vi "main 0.2.vi"() -> ()   [LabVIEW 2020]
uses:
  subvi/Newport ESP301/Newport ESP301.lvlib
  subvi/sp_manip.llb/sp_manip_lib.lvlib
  subvi/sp_manip.llb/tcp_gateway.lvlib
  <vilib>/Utility/file.llb/Write Delimited Spreadsheet (DBL).vi
  subvi/PHOIBOS/DEFINITIONS/DEF_dev_type.ctl
  subvi/PHOIBOS/DEFINITIONS/DEF_dev_state.ctl
  <vilib>/Utility/file.llb/Write Delimited Spreadsheet (I64).vi
panel:
  out "state":T1 items=["Off"=-1, "Standby"=0, "On"=1]
  in  "BasePath 2":path=path "Z:/PESdata"
  out "ESP_con?":bool caption="ESP301"
  out "phoib_con?":bool caption="PHOIBOS"
  out "manip_con?":bool caption="manipulator"
  out "cam_con?":bool caption="camera"
  in  "main_close":bool
  in  "Tab Control":enum32{"Live", "Measure", "Settings", "Devices"}(tab)=enum."Devices"
  out "cam_burst_progress":u8(slide) scale=0.0..200.0
  in  "cam_burstnr":u32 max=1000
  in  "cam_burst":bool
  in  "ESP_delta":dbl
  in  "ESP_+ 2":bool
  in  "ESP_+":bool
  in  "ESP_go":bool
  in  "ESP_dest_t":dbl caption="Delay"
  in  "ESP_dest":dbl caption="Position"
  in  "ESP_set_t0":bool
  in  "phoib_I_6s":dbl=3200.0
  in  "phoib_I_5s":dbl=1400.0
  in  "phoib_I_4s":dbl=4.2
  in  "phoib_I_3s":dbl
  in  "phoib_I_2s":dbl=35.0
  in  "phoib_I_1s":dbl=21.9
  in  "phoib_standby":bool
  in  "phoib_set":bool
  out "phoib_I_6":dbl caption="Screen Voltage"
  out "phoib_I_5":dbl caption="Detctor Voltage"
  out "phoib_I_4":dbl caption="Work Function"
  out "phoib_I_3":dbl caption="Coil Current"
  out "phoib_I_2":dbl caption="Pass Energy"
  out "phoib_I_1":dbl caption="Kinetic Energy"
  out "CCD temp [°C]":i32=-13
  out "electronics temp [°C]":i32=30
  out "Saved Positions":string[][](table)=[["ertwertwert", "-2.299945", "-2.030214", "38.900024", "50.000762", "0.000887", "-97.998082"], ["uztgugt", "-14.999451", "-13.638894", "442.380066", "13.998380", "-1.893758", "-76.305838"], ["asdf", "-14.999451", "-13.638894", "442.380066", "13.998380", "-1.893758", "-76.305838"], ["test3", "-14.999451", "-13.638894", "441.380066", "13.998380", "-1.893758", "-76.305838"]]
  in  "Save Pos":bool
  in  "Load":bool
  in  "Delete":bool
  in  "ManipRel":dbl=1.0
  in  "ManipRel +":bool
  in  "ManipRel -":bool
  in  "manip.rel.select":enum32{"x", "y", "z", "polar", "tilt", "azimut"}(radio)=enum."polar"
  in  "Move Abs":bool
  in  "stop manip":bool
  in  "dest":dbl[](array[numeric])=[0.007141549166819264, -0.009888298846365134, 431.30615234375, 89.00040512814502, 1.109125024699864, -227.9162918846475] caption="destinations" format="%#.5g"
  out "names":string[](array[string])=["x", "y", "z", "polar", "tilt", "azimut"]
  out "pos":dbl[](array[numeric])=[0.007141549166819264, -0.009888298846365134, 431.30615234375, 89.00040512814502, 1.109125024699864, -227.9162918846475] caption="positions" format="%.5f"
  out "Intensity Graph":u16[][](graph)
  in  "Exposure [ms]":u32=20
  in  "Mode":T2(ring)=enum."WideAngleMode"
  in  "VoltageRange":enum16{"3.5kV", "1.5kV", "400V", "100V", "10V"}(ring)=enum."400V"
  out "ESP_pos":dbl caption="Position"
  out "ESP_delay":dbl caption="Delay"
  in  "ESP_t0":dbl caption="Time Zero @"
  in  "V binning":u16(ring)=2 items=["X 1", "X 2", "X 4", "X 8", "X 16", "X 32", "X 64", "X 128", "X 256", "X 512", "X 1024"]
  in  "H binning":u16(ring)=2 items=["X 1", "X 2", "X 4", "X 8"]
  in  "cam_gain":bool
  out "opti_frames":dbl=25.0 caption="#steps_opti"
  out "opti_current_frame":i32=25
  out "Measurement Progress":u8(slide) scale=0.0..100.0
  out "Camera Aquisition":u8(slide) scale=0.0..100.0
  in  "Optimize":bool
  in  "OptiStepSize":dbl=-1.0 caption="Step Size"
  in  "OptiRange":dbl=25.0 caption="Range"
  in  "meas_axis":string(combo)="tilt" caption="Axis"
  in  "meas_avg":i32=60 caption="Frames2Average"
  in  "OptiCancel":bool
  out "#steps_opti":dbl=25.0
  out "current_step_opti":i32=25
  out "ETA":string
  in  "BasePath":path=path "Z:/PESdata"
  in  "Path":path=path "Z:/software/ManipulatorControl/save.txt"
  in  "ROI Bottom":i32=32
  in  "ROI Top":i32=1
  in  "ROI Right":i32=40
  in  "ROI Left":i32=1
  in  "ESP Axis":i32=1 min=1 max=3
  in  "manip_init":bool
  in  "manip_release":bool
  in  "phoib_init":bool
  in  "phoib_release":bool
  in  "ESP_init":bool
  in  "ESP_release":bool
  in  "ESP301 VISA":refnum<visa-resource-name>="COM8"
  in  "cam_boardnr":i32
  in  "cam_init":bool
  in  "cam_release":bool
  out "error out":errorcluster
  out "error out 2":errorcluster
  # "step _ of _"
  # "step _ of _"
  # "manip"
  # "phoib"
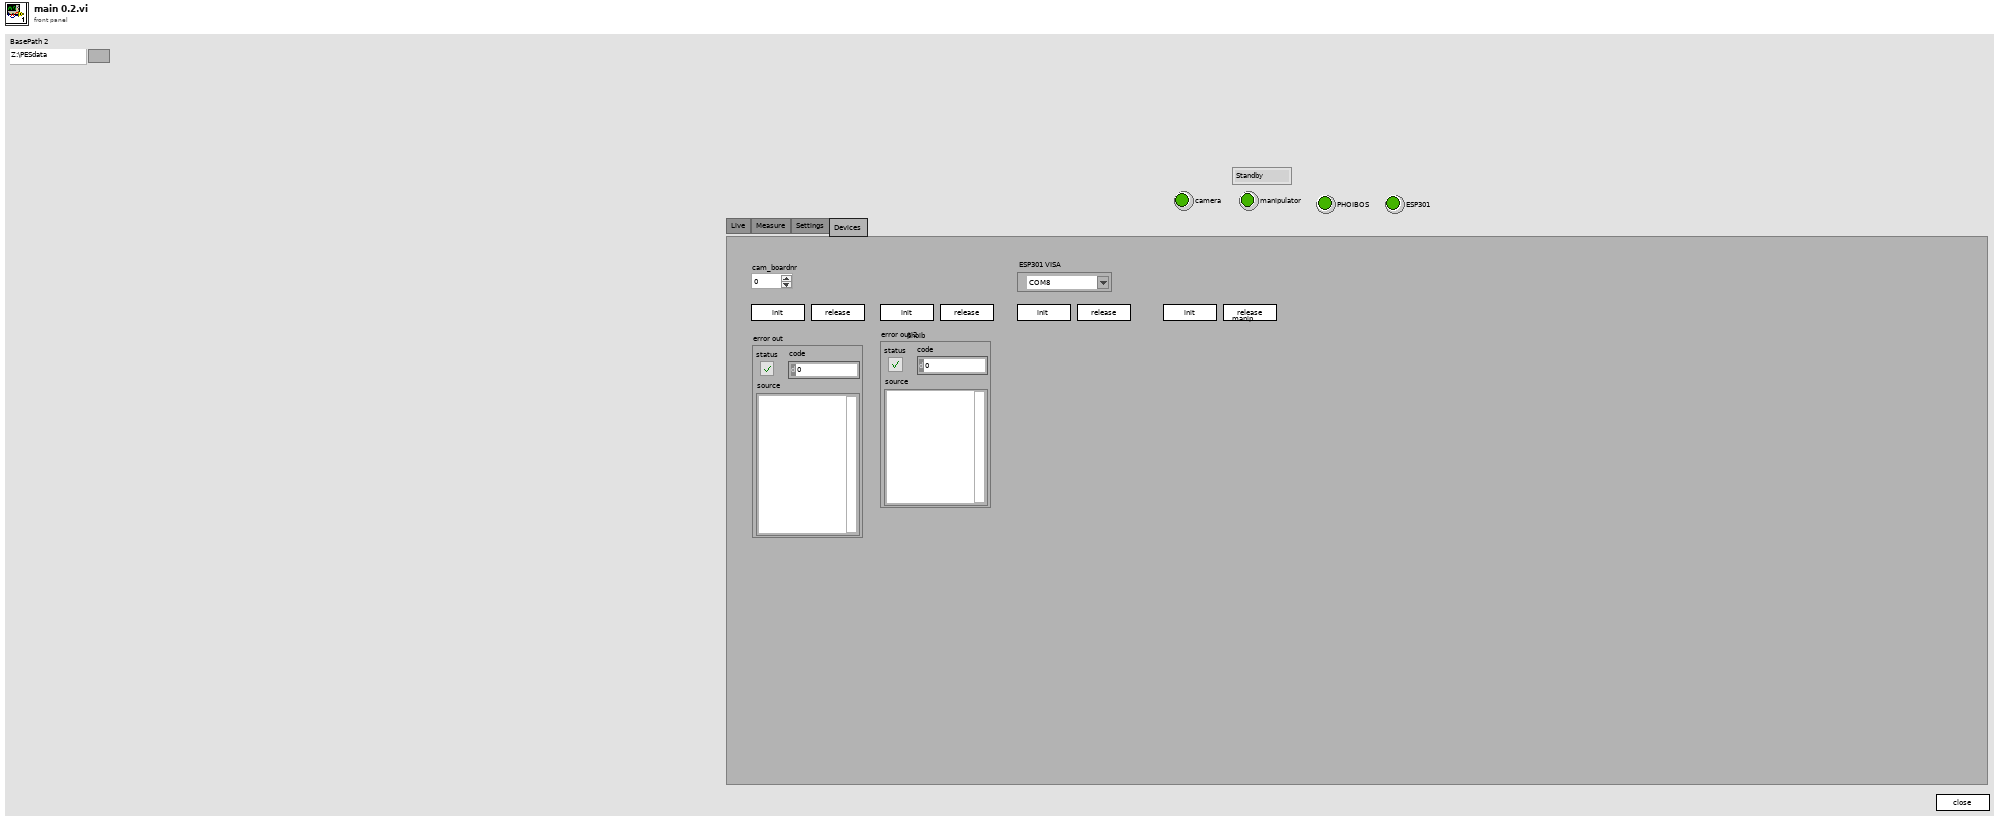
[diagram p1: front panel]
types:
  T1 = typedef "DEF_dev_state.ctl" = i32
  T2 = enum16{"HighMagnification", "MediumMagnification", "LowMagnification", "HighAngularDispersion", "MediumAngularDispersion", "LowAngularDispersion", "WideAngleMode", "LargeArea", "MediumArea", "SmallArea", "HighMagnification2", "SmallArea2", "ImagingMode"}
  T3 = cluster{"Camera type":u32, "Operating mode\nHP & QE / HS & DiCam Pro ":u32, "Frame trigger \n(High Performance and QE only)":u16, "Sequence trigger":u16, "Low Light\n(QE only)":bool, "Gain":bool, "Horzontal\nbinning":u16, "Vertical\nbinning ":u16, "ROI Left":i32, "ROI Right":i32, "ROI Top":i32, "ROI Bottom":i32}
  T4 = enum16{"open", "replace", "create", "open or create", "replace or create", "replace or create with confirmation"}
  T5 = cluster{"Axis_Name":string, "Axis_Type":string, "Axis_Position":dbl, "continous":bool, "moving":bool}[]
  T6 = cluster{"Axis_Name":string, "Axis_Type":string, "Axis_Position":dbl, "continous":bool, "moving":bool}
  T7 = typedef "DEF_dev_type.ctl" = enum32{"devA (analyzer)", "devD (detector)"}
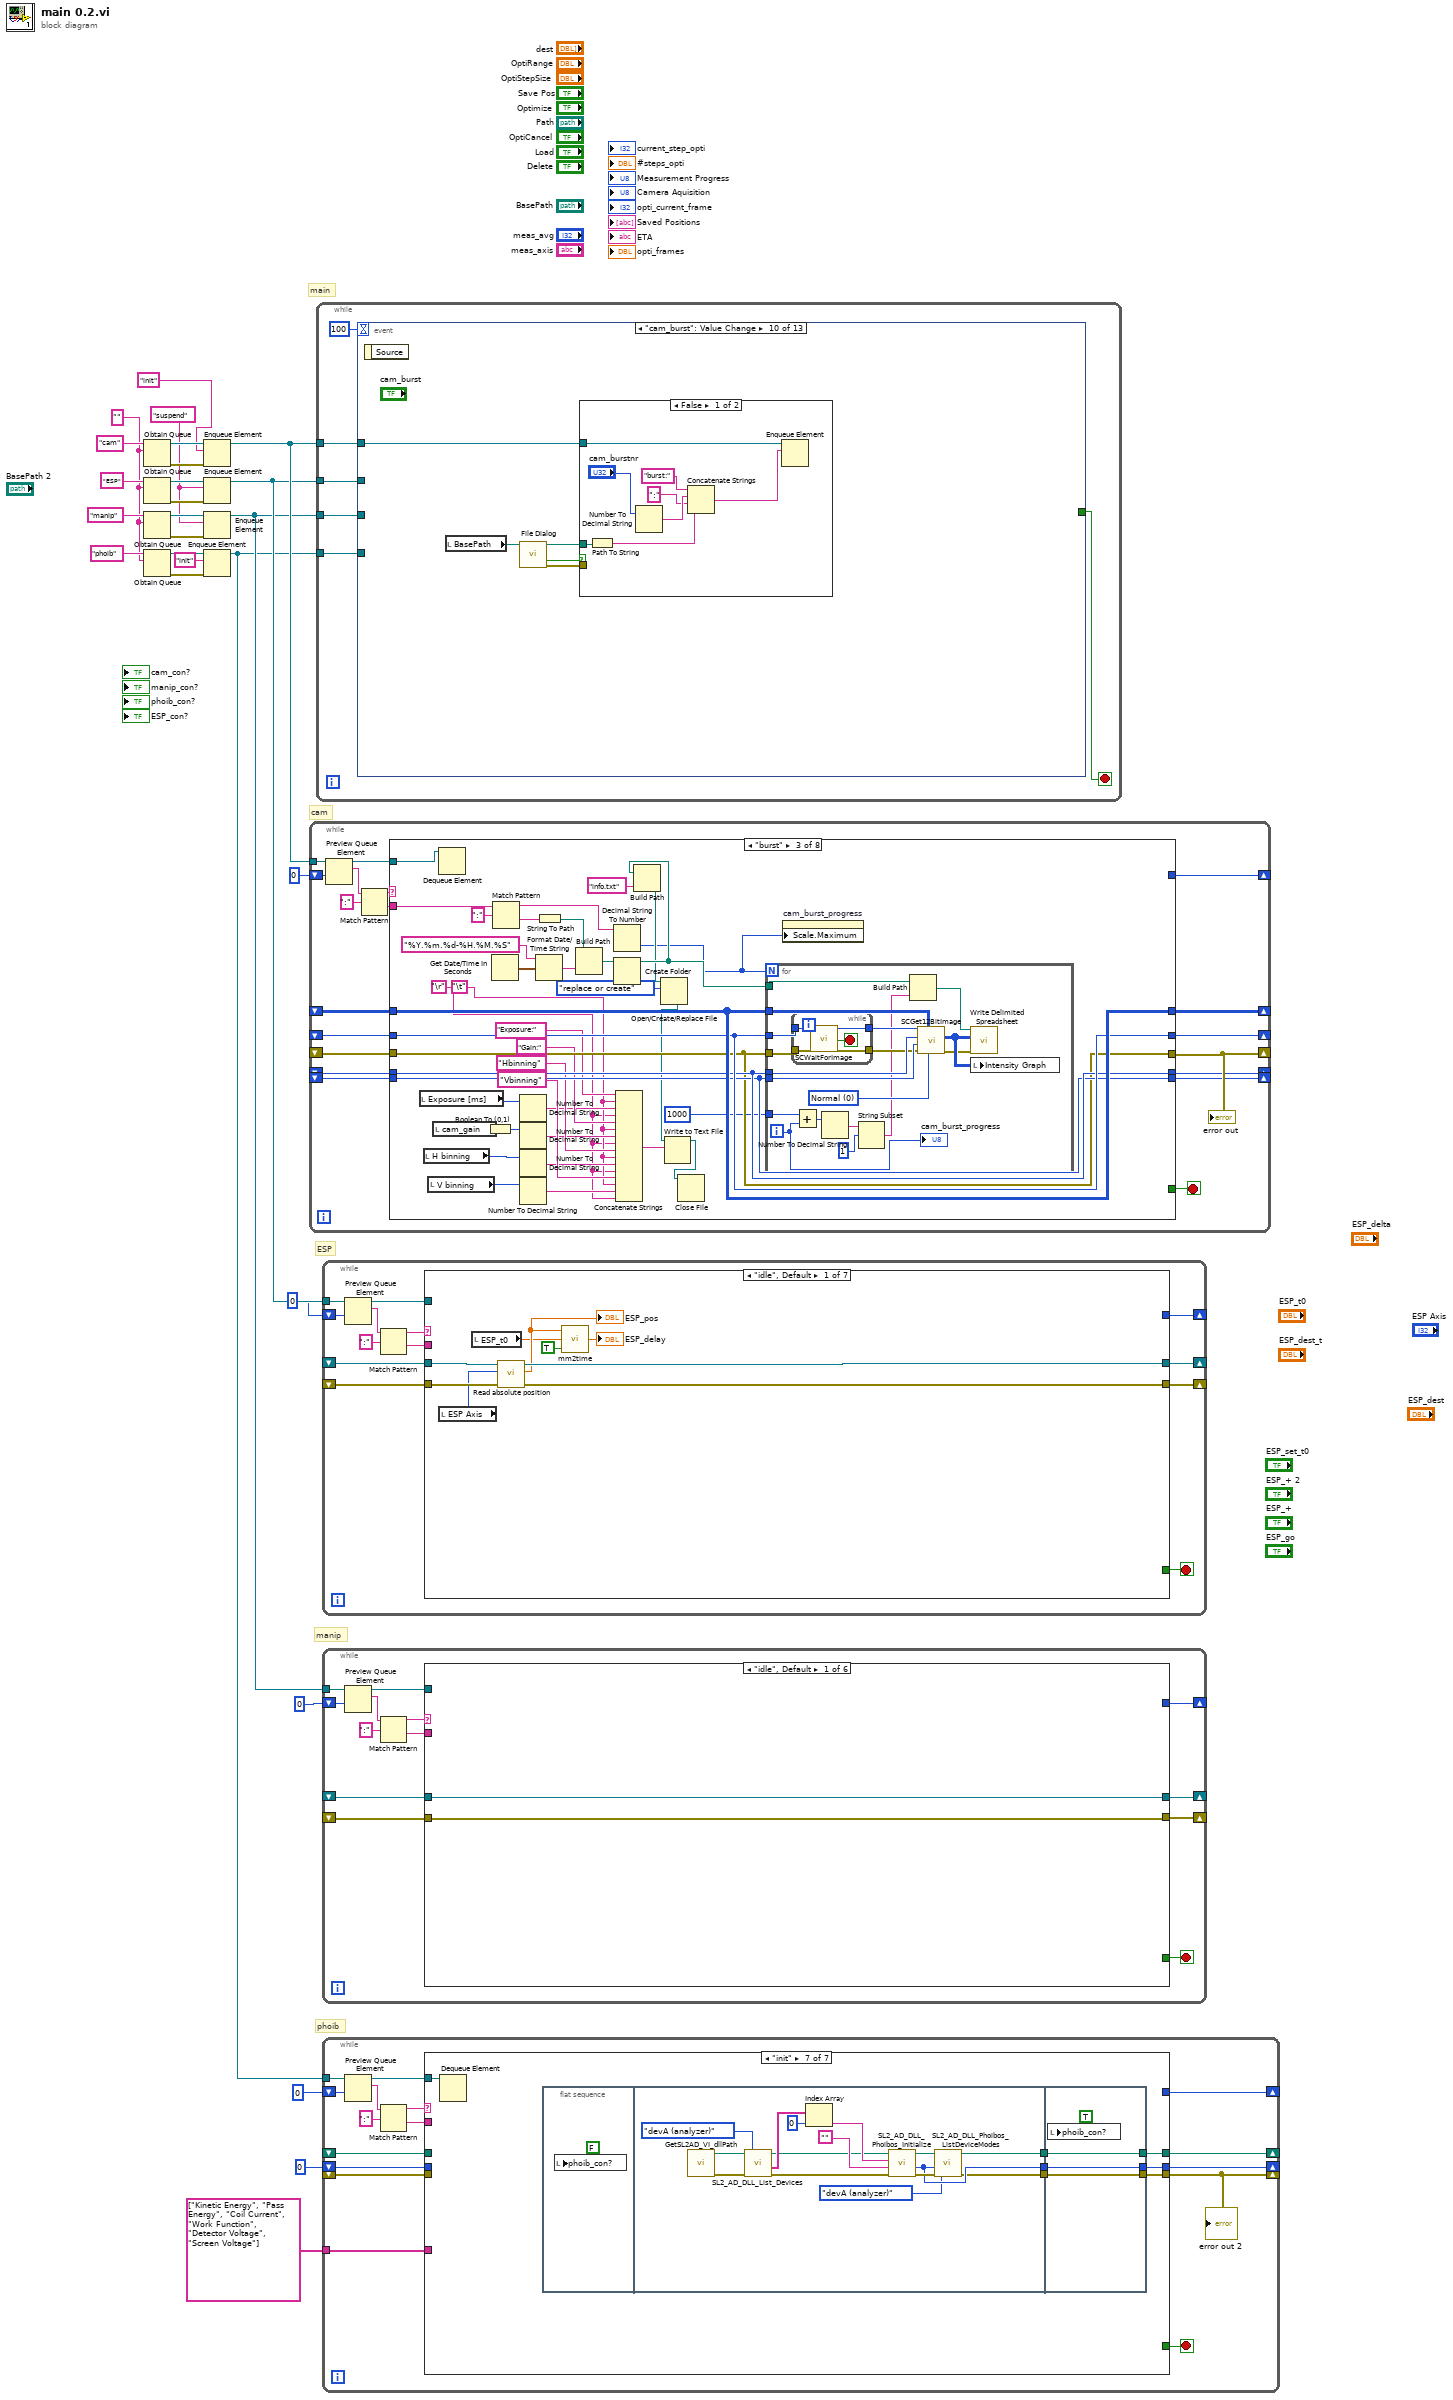
[diagram p0: block diagram]
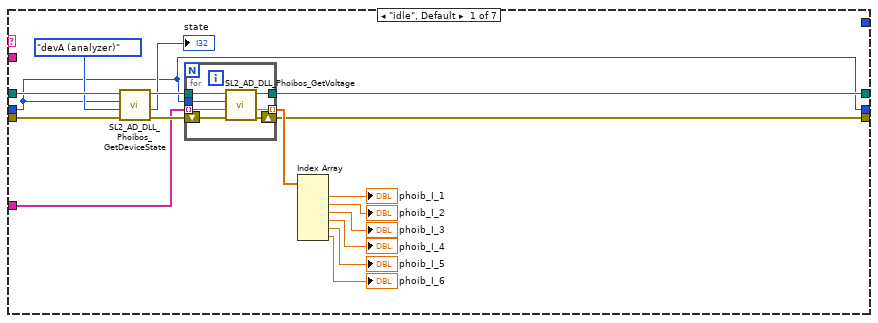
[diagram p2: hidden frame]
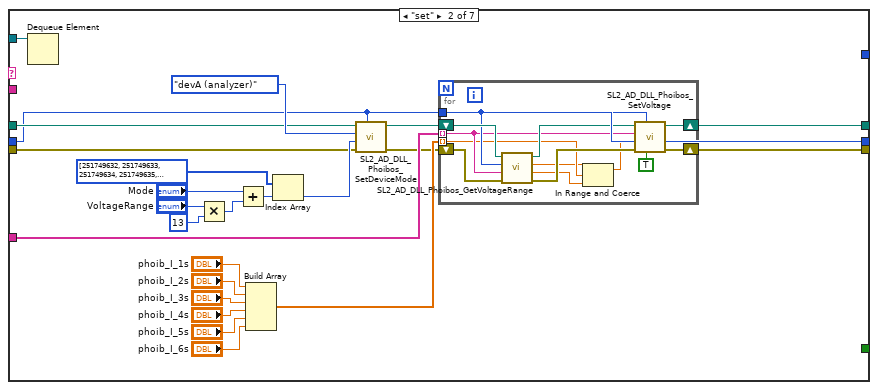
[diagram p3: hidden frame]
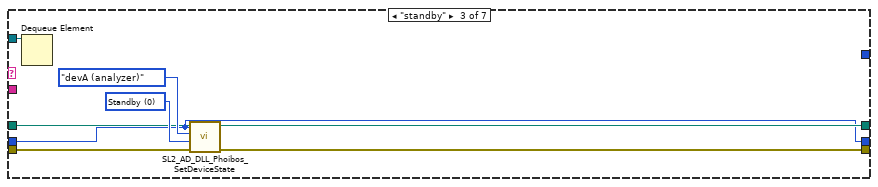
[diagram p4: hidden frame]
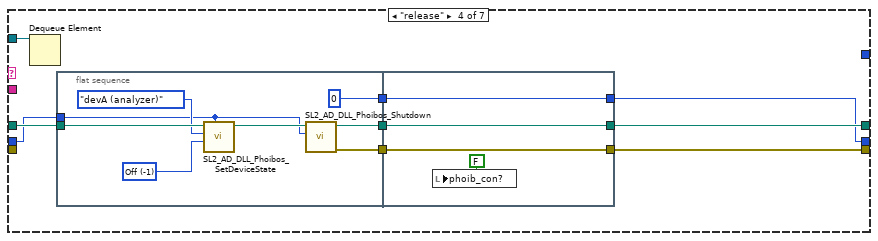
[diagram p5: hidden frame]
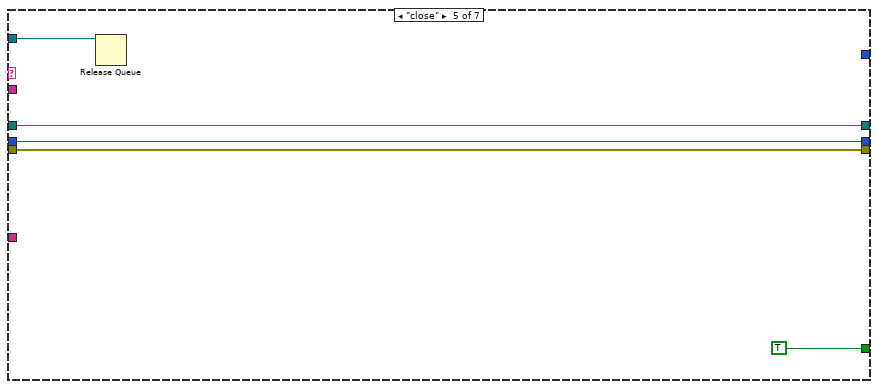
[diagram p6: hidden frame]
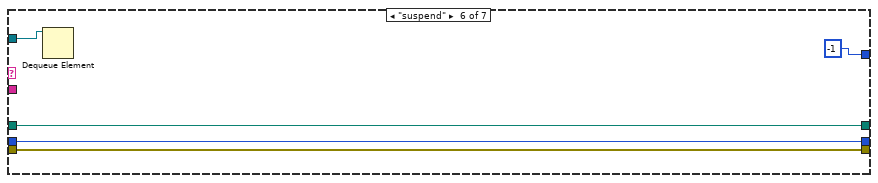
[diagram p7: hidden frame]
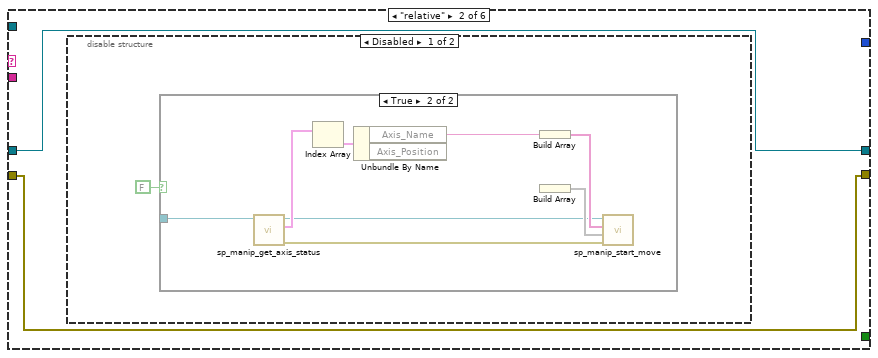
[diagram p8: hidden frame]
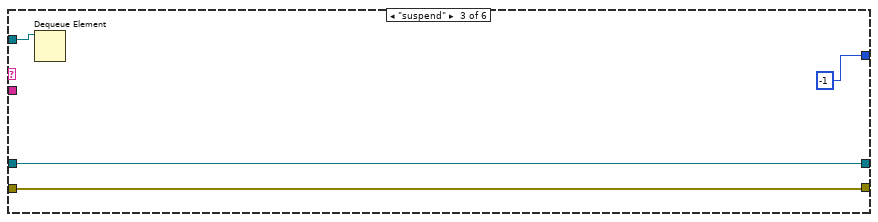
[diagram p11: hidden frame]
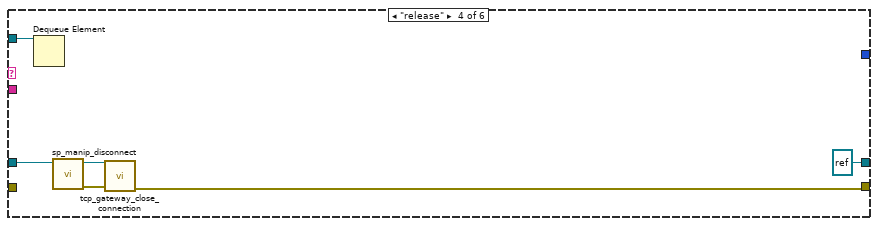
[diagram p12: hidden frame]
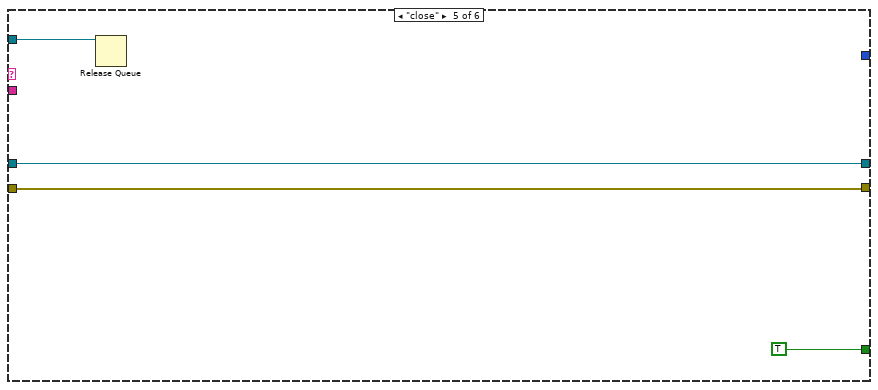
[diagram p13: hidden frame]
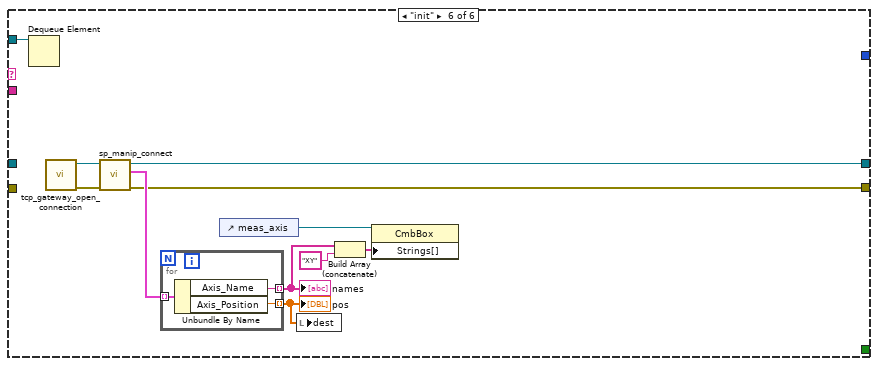
[diagram p14: hidden frame]
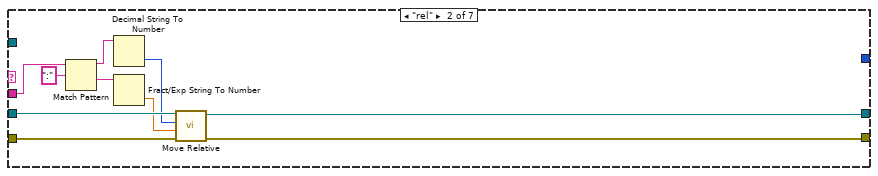
[diagram p15: hidden frame]
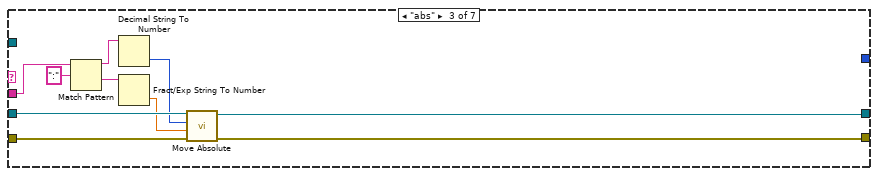
[diagram p16: hidden frame]
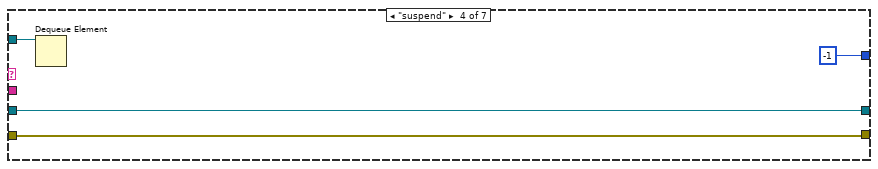
[diagram p17: hidden frame]
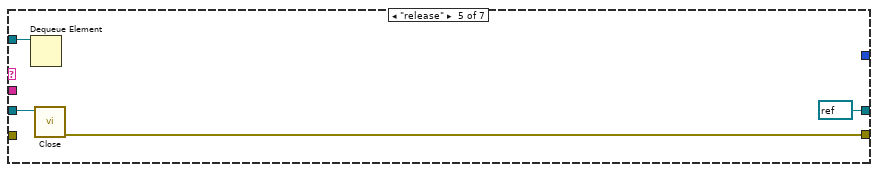
[diagram p18: hidden frame]
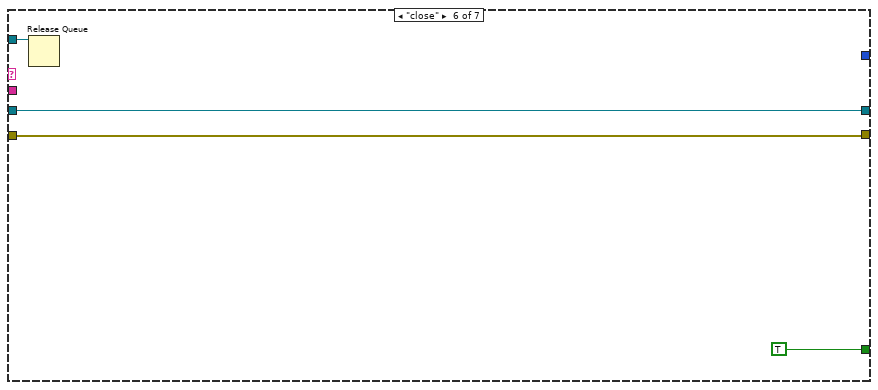
[diagram p19: hidden frame]
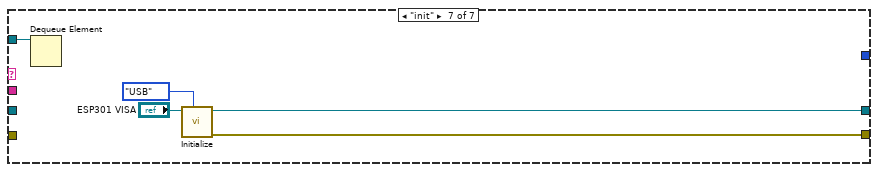
[diagram p20: hidden frame]
diagram:
  w13 = "suspend" ("name (unnamed)")
  w12 = "" ("name (unnamed)")
  # "phoib"
  # "manip"
  # "ESP"
  # "cam"
  # "main"
  n1 = Obtain Queue(name (unnamed)="cam", element data type=w12) -> (queue out=w25:refnum<queue>, error out=w24:errorcluster)  [unwired: 3 in, 1 out]
  n2 = Obtain Queue(name (unnamed)="ESP", element data type=w12) -> (queue out=w21:refnum<queue>, error out=w22:errorcluster)  [unwired: 3 in, 1 out]
  n3 = Obtain Queue(name (unnamed)="manip", element data type=w12) -> (queue out=w18:refnum<queue>, error out=w17:errorcluster)  [unwired: 3 in, 1 out]
  n4 = Obtain Queue(name (unnamed)="phoib", element data type=w12) -> (queue out=w15:refnum<queue>, error out=w16:errorcluster)  [unwired: 3 in, 1 out]
  n5 = Enqueue Element(queue=w25, element="init" ("name (unnamed)"), error in (no error)=w24) -> (queue out=w23:refnum<queue>)  [unwired: 1 in, 2 out]
  n6 = Enqueue Element(queue=w21, element=w13, error in (no error)=w22) -> (queue out=w11:refnum<queue>)  [unwired: 1 in, 2 out]
  n7 = Enqueue Element(queue=w18, element=w13, error in (no error)=w17) -> (queue out=w10:refnum<queue>)  [unwired: 1 in, 2 out]
  n8 = Enqueue Element(queue=w15, element="init", error in (no error)=w16) -> (queue out=w9:refnum<queue>)  [unwired: 1 in, 2 out]
  n9 = while {
    tunnel: w23 -> [w45]
    shift-right: [w39] -> _
    shift-left: _ -> [w38]
    shift-right: [w37] -> _
    shift-left: _ -> [w33]
    shift-right: [w36] -> _
    shift-left: _ -> [w32]
    shift-right: [w35] -> _
    shift-left: _ -> [w31]
    shift-right: [w34] -> _
    shift-left: _ -> [w30]
    shift-right: [w27] -> _
    shift-left: 0 -> [w28]
    stop <- w29 stop-if-true
    n10 = Preview Queue Element(queue=w45, timeout in ms (-1)=w28) -> (queue out=w44:refnum<queue>, element=w43:string)  [unwired: 1 in, 2 out]
    n11 = Match Pattern(string=w43, regular expression=":") -> (before substring=w40:string, after substring=w41:string)  [unwired: 1 in, 2 out]
    n12 = case shown="\"burst\"" w40 {
      tunnel: w44 -> [w54 w77 w123 w168 w179 _ _ w230]
      tunnel: w41 -> [_ _ w136 _ _ _ w206 _]
      tunnel: [u16[][] [] w78 w133 w167 w177 w194 w204 w228] -> w39
      tunnel: w38 -> [_ _ w133 w167 w177 w194 w204 w228]
      tunnel: [w53 w79 w132 u64 0 ("Hout") w176 w185 w203 w227] -> w37
      tunnel: [w55 w80 w129 w162 w175 w188 w202 w226] -> w36
      tunnel: [0 ("Horizontal size") w75 w131 w166 w174 w193 w201 w225] -> w35
      tunnel: [0 ("Vertical size") w74 w130 w165 w173 w192 w200 w224] -> w34
      tunnel: w33 -> [_ w82 w132 w164 w176 w183 w203 w227]
      tunnel: w32 -> [_ w81 w129 _ w175 w182 w213 w226]
      tunnel: w31 -> [_ _ w131 w166 w174 w193 w201 w225]
      tunnel: w30 -> [_ _ w130 w165 w173 w192 w200 w224]
      tunnel: [_ _ _ _ TRUE _ _ _] -> w29
      tunnel: [_ _ _ _ _ _ _ -1] -> w27
      frame "init" {
        n13 = Dequeue Element(queue=w54) -> (queue out=w47:refnum<queue>)  [unwired: 2 in, 3 out]
        n14 = Enqueue Element At Opposite End(queue=w47, element="set") -> ()  [unwired: 2 in, 3 out]
        n15 = flat-sequence {
          tunnel: [w57] -> w52
          tunnel: [w58] -> w51
          tunnel: [w66] -> w53
          tunnel: [w67] -> w55
          tunnel: w52 -> [w67]
          tunnel: w51 -> [w66]
          frame #0 {
            n16 = local write "cam_con?"(FALSE ("cam_con?")) -> ()
          }
          frame #1 {
            n17 = call "SCInitBoard.vi"("boardnr"="cam_boardnr") -> ("Hout"=w61:u32, "error out"=w62:errorcluster)  [unwired: 1 in, 1 out]
            n18 = call "SCSetupCamera.vi"("Handle"=w61, "error in (no error)"=w62) -> ("Hout"=w63:u64, "error out"=w64:errorcluster)  [unwired: 1 out]
            n19 = call "SCStopCOC.vi"("error in (no error)"=w64, "Stop mode"=0, "Handle"=w63) -> ("error out"=w57:errorcluster, "Hout"=w58:u64)
          }
          frame #2 {
            n20 = local write "cam_con?"(TRUE ("cam_con?")) -> ()
          }
        }
      }
      frame "set" {
        w76 = u32 1 ("Operating mode\nHP & QE / HS & DiCam Pro")
        n21 = Dequeue Element(queue=w77) -> ()  [unwired: 2 in, 4 out]
        n22 = Bundle By Name(cluster=cluster{"Delay":dbl, "Exposure ":dbl} {"Delay"=0.0, "Exposure "=0.0} ("Delay and exposure"), "Exposure"="Exposure [ms]") -> (w69:cluster{"Delay":dbl, "Exposure ":dbl})
        n23 = Bundle By Name(cluster=T3 {"Camera type"=0, "Operating mode\nHP & QE / HS & DiCam Pro "=0, "Frame trigger \n(High Performance and QE only)"=0, "Sequence trigger"=0, "Low Light\n(QE only)"=FALSE, "Gain"=FALSE, "Horzontal\nbinning"=0, "Vertical\nbinning "=0, "ROI Left"=1, "ROI Right"=20, "ROI Top"=1, "ROI Bottom"=15} ("Camera controls"), "Operating mode\nHP & QE / HS & DiCam Pro"=w76, "Horzontal\nbinning"="H binning", "Vertical\nbinning"="V binning", "ROI Left"="ROI Left", "ROI Right"="ROI Right", "ROI Top"="ROI Top", "ROI Bottom"="ROI Bottom", "Gain"="cam_gain") -> (w93:T3)
        n24 = call "New delay and exposure forma.vi"("Operating mode\nHP & QE / HS & DiCam Pro"=w76, "Delay and exposure"=w69) -> ("Output table"=w94:string)  [unwired: 3 in]
        n25 = call "SCStopCOC.vi"("error in (no error)"=w81, "Stop mode"=0, "Handle"=w82) -> ("error out"=w98:errorcluster, "Hout"=w97:u64)
        n26 = call "SCSetCoC.vi"("error in (no error)"=w98, "Delay and exposure table"=w94, "Camera controls"=w93, "Handle"=w97) -> ("error out"=w86:errorcluster, "Hout"=w85:u64)  [unwired: 1 out]
        n27 = call "SCGetImageSize.vi"("Handle"=w85, "error in (no error)"=w86) -> ("Hout"=w84:u64, "error out"=w83:errorcluster, "Horizontal size"=w75:i32, "Vertical size"=w74:i32)  [unwired: 2 out]
        n28 = Initialize Array(u16 0 ("dimension size"), w74, w75) -> (w78:u16[][])
        n29 = call "SCRun.vi"("error in (no error)"=w83, "Run mode"=0, "Handle"=w84) -> ("error out"=w80:errorcluster, "Hout"=w79:u64)  [unwired: 1 out]
      }
      frame "burst" {
        w100 = "\r"
        w101 = "\t"
        n30 = local read "Exposure [ms]"() -> (w109:u32)
        n31 = local read "H binning"() -> (w111:u16)
        n32 = local read "V binning"() -> (w112:u16)
        n33 = local read "cam_gain"() -> (w110:bool)
        n34 = Dequeue Element(queue=w123) -> ()  [unwired: 2 in, 4 out]
        n35 = Boolean To (0,1)(Boolean=w110) -> (0, 1=w113:i16)
        n36 = Get Date/Time In Seconds() -> (seconds since 1Jan1904=w128:timestamp)
        n37 = Match Pattern(string=w136, regular expression=":") -> (before substring=w135:string, after substring=w134:string)  [unwired: 1 in, 2 out]
        n38 = Number To Decimal String(number=w109) -> (decimal integer string=w115:string)  [unwired: 1 in]
        n39 = Number To Decimal String(number=w113) -> (decimal integer string=w117:string)  [unwired: 1 in]
        n40 = Number To Decimal String(number=w111) -> (decimal integer string=w119:string)  [unwired: 1 in]
        n41 = Number To Decimal String(number=w112) -> (decimal integer string=w121:string)  [unwired: 1 in]
        n42 = String To Path(string=w134) -> (path=w126:path)
        n43 = Format Date/Time String(time format string (%c)="%Y.%m.%d-%H.%M.%S", seconds (now)=w128) -> (date/time string=w125:string)  [unwired: 1 in]
        n44 = Build Path(base path=w126, name or relative path=w125) -> (appended path=w124:path)
        n45 = Decimal String To Number(string=w135) -> (number=w99:i32)  [unwired: 2 in, 1 out]
        n46 = Create Folder(path (use dialog)=w124) -> (created path=w104:path)  [unwired: 2 in, 2 out]
        n47 = Concatenate Strings("Exposure:", w101, w115, w100, "Gain:", w101, w117, w100, "Hbinning", w101, w119, w100, "Vbinning", w101, w121, w100) -> (w108:string)
        n48 = Build Path(base path=w104, name or relative path="info.txt") -> (appended path=w103:path)
        n49 = Open/Create/Replace File(file path (use dialog)=w103, operation (0:open)=T4."replace or create") -> (refnum out=w106:refnum<file>)  [unwired: 4 in, 2 out]
        n50 = Write to Text File(file (use dialog)=w106, text=w108) -> (refnum out=w107:refnum<file>)  [unwired: 2 in, 2 out]
        n51 = Close File(refnum=w107) -> ()  [unwired: 1 in, 2 out]
        n52 = for {
          N: w99 -> [_]
          tunnel: w133 -> [w154]
          tunnel: w132 -> [w151]
          tunnel: w129 -> [w150]
          tunnel: w131 -> [w153]
          tunnel: w130 -> [w152]
          tunnel: w104 -> [w145]
          tunnel: 1000 ("x") -> [w143]
          i -> [w138]
          w155 = 0 items=["Normal", "Upside down"] ("mode")
          n53 = while {
            tunnel: [w159] -> w148
            tunnel: [w158] -> w149
            tunnel: w151 -> [w157]
            tunnel: w150 -> [w156]
            stop <- w160 stop-if-true
            n54 = call "SCWaitForImage.vi"("Handle"=w157, "error in (no error)"=w156) -> ("Hout"=w158:u64, "Image Valid"=w160:bool, "error out"=w159:errorcluster)  [unwired: 15 in]
          }
          n55 = Add(x=w143, y=w138) -> (x+y=w142:i32)
          n56 = Number To Decimal String(number=w142) -> (decimal integer string=w141:string)  [unwired: 1 in]
          n57 = String Subset(string=w141, offset (0)=1) -> (substring=w139:string)  [unwired: 1 in]
          n58 = Build Path(base path=w145, name or relative path=w139) -> (appended path=w144:path)
          n59 = call "SCGet12BitImage.vi"("mode"=w155, "Input array"=w154, "error in (no error)"=w148, "Vertical size"=w152, "Horizontal size"=w153, "Handle"=w149) -> ("error out"=w146:errorcluster, "imgdata"=w147:u16[][])  [unwired: 1 in, 1 out]
          n60 = call-poly <vilib>:"Write Delimited Spreadsheet.vi"("file path (dialog if empty)"=w144, "2D data"=w147, "error in (no error)"=w146) -> ()  [unwired: 11 in, 2 out]
          n61 = local write "Intensity Graph"(w147) -> ()
          "cam_burst_progress" <- w138
        }
        n62 = property on="cam_burst_progress" class="Slide (strict)"("Scale.Maximum"=w99) -> ()  [unwired: 2 in, 2 out]
      }
      frame "release" {
        n63 = Dequeue Element(queue=w168) -> ()  [unwired: 2 in, 4 out]
        n64 = flat-sequence {
          tunnel: w164 -> [w170]
          tunnel: [w169] -> w161
          tunnel: [w172] -> w162
          tunnel: w161 -> [w172]
          frame #0 {
            n65 = call "SCCloseBoard.vi"("Handle"=w170) -> ("error out"=w169:errorcluster)  [unwired: 1 in, 2 out]
          }
          frame #1 {
            n66 = local write "cam_con?"(FALSE ("cam_con?")) -> ()
          }
        }
      }
      frame "close" {
        n67 = Release Queue(queue=w179) -> ()  [unwired: 2 in, 3 out]
      }
      frame "idle", Default {
        w191 = 0 items=["Normal", "Upside down"] ("mode")
        n68 = while {
          tunnel: [w198] -> w180
          tunnel: [w197] -> w181
          tunnel: w183 -> [w196]
          tunnel: w182 -> [w195]
          stop <- w199 stop-if-true
          n69 = call "SCWaitForImage.vi"("Handle"=w196, "error in (no error)"=w195) -> ("Hout"=w197:u64, "Image Valid"=w199:bool, "error out"=w198:errorcluster)  [unwired: 15 in]
        }
        n70 = call "SCGet12BitImage.vi"("mode"=w191, "Input array"=w194, "error in (no error)"=w180, "Vertical size"=w192, "Horizontal size"=w193, "Handle"=w181) -> ("error out"=w189:errorcluster, "imgdata"=→"Intensity Graph":u16[][], "Hout"=w190:u64)  [unwired: 1 in]
        n71 = call "SCGetStatus.vi"("Handle"=w190, "error in (no error)"=w189) -> ("Hout"=w185:u64, "Electronics temperature"=→"electronics temp [°C]":i32, "CCD temperature"=→"CCD temp [°C]":i32, "error out"=w188:errorcluster)  [unwired: 2 out]
      }
      frame "snap" {
        n72 = local read "BasePath 2"() -> (w215:path)
        n73 = local read "meas_avg"() -> (w210:i32)
        n74 = Initialize Array(u32 0 ("element"), w201, w200) -> (w212:u32[][])
        n75 = Build Path(base path=w215, name or relative path=w206) -> (appended path=w205:path)
        n76 = for {
          N: w210 -> [_]
          tunnel: w201 -> [w223]
          tunnel: w200 -> [w222]
          tunnel: w204 -> [w220]
          shift-right: [w217] -> w211
          shift-left: w212 -> [w219]
          shift-right: [w216] -> w202
          shift-left: w213 -> [w221]
          n77 = call "SCGet12BitImage.vi"("Input array"=w220, "error in (no error)"=w221, "Vertical size"=w222, "Horizontal size"=w223) -> ("error out"=w216:errorcluster, "imgdata"=w218:u16[][])  [unwired: 3 in, 1 out]
          n78 = Add(x=w218, y=w219) -> (x+y=w217:u32[][])
        }
        n79 = Divide(x=w211, y=w210) -> (x/y=w209:dbl[][])
        n80 = call-poly <vilib>:"Write Delimited Spreadsheet.vi"("file path (dialog if empty)"=w205, "format (%.3f)"="%d", "2D data"=w209, "transpose? (no:F)"=TRUE ("transpose? (F)")) -> ()  [unwired: 10 in, 2 out]
      }
      frame "suspend" {
        n81 = Dequeue Element(queue=w230) -> ()  [unwired: 2 in, 4 out]
      }
    }
    "error out" <- w36
  }
  n82 = while {
    tunnel: w23 -> [w234]
    tunnel: w11 -> [w233]
    tunnel: w10 -> [w232]
    tunnel: w9 -> [w231]
    stop <- w236 stop-if-true
    n83 = event shown="[9] \"cam_burst\": Value Change" {
      selector: _ -> [_ _ _ _ _ _ _ _ _ _ _ _ _]
      dyn-events: _ -> [_ _ _ _ _ _ _ _ _ _ _ _ _]
      timeout: 100 -> [_ _ _ _ _ _ _ _ _ _ _ _ _]
      tunnel: [_ TRUE _ _ _ _ _ _ _ _ _ _ _] -> w236
      tunnel: w234 -> [_ w246 w249 _ _ _ _ _ w275 w276 _ _ _]
      tunnel: w233 -> [_ w245 _ w253 _ _ _ _ _ _ _ _ _]
      tunnel: w232 -> [_ w244 _ _ w259 _ _ _ _ _ _ _ _]
      tunnel: w231 -> [_ w243 _ _ _ w265 w271 w272 _ _ _ _ _]
      event Timeout {
        n84 = event-data() -> ()  [unwired: 1 in, 1 out]
      }
      event "main_close": Value Change {
        w237 = "close" ("element")
        w242 = "release" ("element")
        n85 = event-data() -> ()  [unwired: 1 in, 1 out]
        n86 = Enqueue Element(queue=w246, element=w242) -> (queue out=w241:refnum<queue>)  [unwired: 2 in, 2 out]
        n87 = Enqueue Element(queue=w245, element=w242) -> (queue out=w240:refnum<queue>)  [unwired: 2 in, 2 out]
        n88 = Enqueue Element(queue=w244, element=w242) -> (queue out=w239:refnum<queue>)  [unwired: 2 in, 2 out]
        n89 = Enqueue Element(queue=w243, element=w242) -> (queue out=w238:refnum<queue>)  [unwired: 2 in, 2 out]
        n90 = Enqueue Element(queue=w241, element=w237) -> ()  [unwired: 2 in, 3 out]
        n91 = Enqueue Element(queue=w240, element=w237) -> ()  [unwired: 2 in, 3 out]
        n92 = Enqueue Element(queue=w239, element=w237) -> ()  [unwired: 2 in, 3 out]
        n93 = Enqueue Element(queue=w238, element=w237) -> ()  [unwired: 2 in, 3 out]
      }
      event "cam_release", "cam_init": Value Change {
        n94 = event-data() -> ()  [unwired: 1 in, 2 out]
        n95 = Select(t="init" ("name (unnamed)"), s="cam_init", f="release" ("name (unnamed)")) -> (s? t:f=w248:string)
        n96 = Enqueue Element(queue=w249, element=w248) -> ()  [unwired: 2 in, 3 out]
      }
      event "ESP_release", "ESP_init": Value Change {
        n97 = event-data() -> ()  [unwired: 1 in, 2 out]
        n98 = Select(t="init" ("name (unnamed)"), s="ESP_init", f="release" ("name (unnamed)")) -> (s? t:f=w257:string)
        n99 = Enqueue Element(queue=w253, element=w257) -> ()  [unwired: 2 in, 3 out]
      }
      event "manip_init", "manip_release": Value Change {
        n100 = event-data() -> ()  [unwired: 1 in, 2 out]
        n101 = Flush Queue(queue=w259) -> (queue out=w258:refnum<queue>)  [unwired: 1 in, 2 out]
        n102 = Select(t="init" ("name (unnamed)"), s="manip_init", f="release" ("name (unnamed)")) -> (s? t:f=w261:string)
        n103 = Enqueue Element(queue=w258, element=w261) -> ()  [unwired: 2 in, 3 out]
      }
      event "phoib_release", "phoib_init": Value Change {
        n104 = event-data() -> ()  [unwired: 1 in, 2 out]
        n105 = Flush Queue(queue=w265) -> (queue out=w264:refnum<queue>)  [unwired: 1 in, 2 out]
        n106 = Select(t="init" ("name (unnamed)"), s="phoib_init", f="release" ("name (unnamed)")) -> (s? t:f=w267:string)
        n107 = Enqueue Element(queue=w264, element=w267) -> ()  [unwired: 2 in, 3 out]
      }
      event "phoib_standby": Value Change {
        n108 = event-data() -> ()  [unwired: 1 in, 2 out]
        n109 = Enqueue Element(queue=w271, element="standby") -> ()  [unwired: 2 in, 3 out]
      }
      event "phoib_set": Value Change {
        n110 = event-data() -> ()  [unwired: 1 in, 2 out]
        n111 = Enqueue Element(queue=w272, element="set") -> ()  [unwired: 2 in, 3 out]
      }
      event "ROI Left", "ROI Right", "ROI Top", "ROI Bottom", "Exposure [ms]", "V binning", "H binning", "cam_gain": Value Change {
        n112 = event-data() -> ()  [unwired: 1 in, 6 out]
        n113 = Enqueue Element(queue=w275, element="set") -> ()  [unwired: 2 in, 3 out]
      }
      event "cam_burst": Value Change {
        n114 = event-data() -> ()  [unwired: 1 in, 1 out]
        n115 = local read "BasePath"() -> (w280:path)
        n116 = call "File Dialog"("start path"=w280) -> ("selected path"=w278:path, "cancelled"=w279:bool, "error out"=w277:errorcluster)  [unwired: 11 in, 1 out]
        n117 = case shown="False" w279 {
          tunnel: w278 -> [w283 _]
          tunnel: w277 -> [_ _]
          tunnel: w276 -> [w288 _]
          frame False {
            n118 = Path To String(path=w283) -> (string=w282:string)
            n119 = Number To Decimal String(number="cam_burstnr") -> (decimal integer string=w285:string)  [unwired: 1 in]
            n120 = Concatenate Strings("burst:" ("string"), w285, ":" ("string"), w282) -> (w281:string)
            n121 = Enqueue Element(queue=w288, element=w281) -> ()  [unwired: 2 in, 3 out]
          }
          frame True {
          }
        }
      }
      event "Move Abs": Value Change {
        n122 = event-data() -> ()  [unwired: 1 in, 1 out]
      }
      event "ManipRel +", "ManipRel -": Value Change {
        n123 = event-data() -> ()  [unwired: 1 in, 2 out]
        n124 = Negate(x="ManipRel") -> (-x=w290:dbl)
        n125 = Select(t=w290, s="ManipRel -", f="ManipRel") -> ()  [unwired: 1 out]
      }
      event "stop manip": Value Change {
        n126 = event-data() -> ()  [unwired: 1 in, 1 out]
      }
    }
  }
  n127 = while {
    tunnel: w11 -> [w299]
    shift-right: [w297] -> _
    shift-left: _ -> [w295]
    shift-right: [w296] -> _
    shift-left: _ -> [w294]
    shift-right: [w292] -> _
    shift-left: 0 -> [w293]
    stop <- w298 stop-if-true
    n128 = Preview Queue Element(queue=w299, timeout in ms (-1)=w293) -> (queue out=w302:refnum<queue>, element=w303:string)  [unwired: 1 in, 2 out]
    n129 = Match Pattern(string=w303, regular expression=":") -> (before substring=w301:string, after substring=w300:string)  [unwired: 1 in, 2 out]
    n130 = case shown="\"idle\", Default" w301 {
      tunnel: w302 -> [_ _ _ w337 w338 w345 w350]
      tunnel: w300 -> [_ w318 w330 _ _ _ _]
      tunnel: [_ _ _ _ _ TRUE _] -> w298
      tunnel: [w311 w320 w326 w335 refnum<visa-resource-name> refnum ("VISA resource name out") w342 w347] -> w297
      tunnel: [w310 w321 w327 w334 w340 w343 w346] -> w296
      tunnel: w295 -> [w313 w323 w328 w335 w341 w342 _]
      tunnel: w294 -> [w312 w322 w329 w334 _ w343 _]
      tunnel: [_ _ _ -1 _ _ _] -> w292
      frame "idle", Default {
        n131 = local read "ESP Axis"() -> (w305:i32)
        n132 = local read "ESP_t0"() -> (w308:dbl)
        n133 = call "Read absolute position.vi"("error in (no error)"=w312, "Axis (1)"=w305, "VISA resource name"=w313) -> ("error out"=w310:errorcluster, "Position (units)"=w309:dbl, "VISA resource name out"=w311:refnum<visa-resource-name>)  [unwired: 2 in]
        "ESP_pos" <- w309
        n134 = call "mm2time.vi"("fs?"=TRUE, "Offset (mm)"=w308, "distance (mm)"=w309) -> ("time in fs/ps seconds"=→"ESP_delay":dbl)
      }
      frame "rel" {
        n135 = Match Pattern(string=w318, regular expression=":") -> (before substring=w317:string, after substring=w316:string)  [unwired: 1 in, 2 out]
        n136 = Decimal String To Number(string=w317) -> (number=w315:i32)  [unwired: 2 in, 1 out]
        n137 = Fract/Exp String To Number(string=w316) -> (number=w314:dbl)  [unwired: 3 in, 1 out]
        n138 = call "Move Relative.vi"("error in (no error)"=w322, "Position (0 units)"=w314, "Axis (1)"=w315, "VISA resource name"=w323) -> ("error out"=w321:errorcluster, "VISA resource name out"=w320:refnum<visa-resource-name>)  [unwired: 2 in]
      }
      frame "abs" {
        n139 = Match Pattern(string=w330, regular expression=":") -> (before substring=w332:string, after substring=w331:string)  [unwired: 1 in, 2 out]
        n140 = Decimal String To Number(string=w332) -> (number=w325:i32)  [unwired: 2 in, 1 out]
        n141 = Fract/Exp String To Number(string=w331) -> (number=w324:dbl)  [unwired: 3 in, 1 out]
        n142 = call "Move Absolute.vi"("error in (no error)"=w329, "Position (0 units)"=w324, "Axis (1)"=w325, "VISA resource name"=w328) -> ("error out"=w327:errorcluster, "VISA resource name out"=w326:refnum<visa-resource-name>)  [unwired: 2 in]
      }
      frame "suspend" {
        n143 = Dequeue Element(queue=w337) -> ()  [unwired: 2 in, 4 out]
      }
      frame "release" {
        n144 = Dequeue Element(queue=w338) -> ()  [unwired: 2 in, 4 out]
        n145 = call "Close.vi"("VISA resource name"=w341) -> ("error out"=w340:errorcluster)  [unwired: 10 in]
      }
      frame "close" {
        n146 = Release Queue(queue=w345) -> ()  [unwired: 2 in, 3 out]
      }
      frame "init" {
        n147 = Dequeue Element(queue=w350) -> ()  [unwired: 2 in, 4 out]
        n148 = call "Initialize.vi"("VISA resource name"="ESP301 VISA", "Serial Link (RS232)"=enum16{"RS232", "USB"}."USB") -> ("VISA resource name out"=w347:refnum<visa-resource-name>, "error out"=w346:errorcluster)  [unwired: 7 in]
      }
    }
  }
  n149 = while {
    tunnel: w10 -> [w358]
    shift-right: [w356] -> _
    shift-left: _ -> [w354]
    shift-right: [w355] -> _
    shift-left: _ -> [w353]
    shift-right: [w351] -> _
    shift-left: 0 -> [w352]
    stop <- w357 stop-if-true
    n150 = Preview Queue Element(queue=w358, timeout in ms (-1)=w352) -> (queue out=w361:refnum<queue>, element=w362:string)  [unwired: 1 in, 2 out]
    n151 = Match Pattern(string=w362, regular expression=":") -> (before substring=w360:string, after substring=w359:string)  [unwired: 1 in, 2 out]
    n152 = case shown="\"idle\", Default" w360 {
      tunnel: w361 -> [_ _ w379 w383 w392 w403]
      tunnel: w359 -> [_ _ _ _ _ _]
      tunnel: [_ _ _ _ TRUE _] -> w357
      tunnel: [w365 w367 w381 refnum<k5> refnum ("gateway_connection out") w390 w394] -> w356
      tunnel: [w364 w366 w380 w385 w389 w393] -> w355
      tunnel: w354 -> [w365 w367 w381 w387 w390 _]
      tunnel: w353 -> [w364 w366 w380 _ w389 _]
      tunnel: [_ _ -1 _ _ _] -> w351
      frame "idle", Default {
      }
      frame "relative" {
        n153 = disable-structure shown="Disabled" {
          frame Disabled {
            n154 = case shown="True" FALSE {
              tunnel: [_ w377] -> w369
              frame False {
              }
              frame True {
                n155 = call "sp_manip_get_axis_status.vi"("gateway_connection"=w377) -> ("error out"=w372:errorcluster, "axis_out"=w376:T5, "gateway_connection out"=w370:refnum<k5>)  [unwired: 6 in, 2 out]
                n156 = Index Array(array=w376) -> (element=w375:T6, index=w378:i32)
                n157 = Unbundle By Name(w375) -> ("Axis_Name"=w371:string)  [unwired: 1 out]
                n158 = Build Array(w371) -> (w374:string[])
                n159 = Build Array() -> (w373:void[])  [unwired: 1 in]
                n160 = call "sp_manip_start_move.vi"("error in"=w372, "target positions"=w373, "axis names"=w374, "gateway_connection"=w370) -> ()  [unwired: 4 in, 4 out]
              }
            }
          }
          frame Enabled {
          }
        }
      }
      frame "suspend" {
        n161 = Dequeue Element(queue=w379) -> ()  [unwired: 2 in, 4 out]
      }
      frame "release" {
        n162 = Dequeue Element(queue=w383) -> ()  [unwired: 2 in, 4 out]
        n163 = call "sp_manip_disconnect.vi"("gateway_connection"=w387) -> ("error out"=w386:errorcluster, "gateway_connection_out"=w388:refnum<k5>)  [unwired: 7 in, 2 out]
        n164 = call "tcp_gateway_close_connection.vi"("error in"=w386, "server_connection"=w388) -> ("error out"=w385:errorcluster)  [unwired: 5 in]
      }
      frame "close" {
        n165 = Release Queue(queue=w392) -> ()  [unwired: 2 in, 3 out]
      }
      frame "init" {
        n166 = Dequeue Element(queue=w403) -> ()  [unwired: 2 in, 4 out]
        n167 = call "tcp_gateway_open_connection.vi"() -> ("gateway_connection"=w398:refnum<k5>, "error out"=w397:errorcluster)  [unwired: 5 in, 3 out]
        n168 = call "sp_manip_connect.vi"("error in"=w397, "gateway_connection"=w398) -> ("error out"=w393:errorcluster, "axis_out"=w396:T5, "gateway_connection out"=w394:refnum<k5>)  [unwired: 5 in, 2 out]
        n169 = for {
          tunnel: w396 -> [w406] mode=indexing
          tunnel: [w405] -> w401 mode=indexing
          tunnel: [w404] -> w402 mode=indexing
          n170 = Unbundle By Name(w406) -> ("Axis_Name"=w405:string, "Axis_Position"=w404:dbl)
        }
        "names" <- w401
        "pos" <- w402
        n171 = control-ref of="meas_axis"() -> (w395:refnum<vi>)
        n172 = local write "dest"(w402) -> ()
        n173 = Build Array (concatenate)(w401, "XY") -> (w399:string[])
        n174 = property on="Property Node" class="CmbBox"(reference=w395, "Strings[]"=w399) -> ()  [unwired: 1 in, 2 out]
      }
    }
  }
  n175 = while {
    tunnel: w9 -> [w417]
    shift-right: [w414] -> _
    shift-left: 0 -> [w415]
    shift-right: [w413] -> _
    shift-left: _ -> [w412]
    shift-right: [w411] -> _
    shift-left: _ -> [w410]
    shift-right: [w409] -> _
    shift-left: u32 0 ("pHandle") -> [w408]
    tunnel: string[] ["Kinetic Energy", "Pass Energy", "Coil Current", "Work Function", "Detector Voltage", "Screen Voltage"] -> [w407]
    stop <- w416 stop-if-true
    n176 = Preview Queue Element(queue=w417, timeout in ms (-1)=w415) -> (queue out=w420:refnum<queue>, element=w421:string)  [unwired: 1 in, 2 out]
    n177 = Match Pattern(string=w421, regular expression=":") -> (before substring=w419:string, after substring=w418:string)  [unwired: 1 in, 2 out]
    n178 = case shown="\"init\"" w419 {
      tunnel: w420 -> [_ w468 w484 w500 w517 w521 w529]
      tunnel: w418 -> [_ _ _ _ _ _ _]
      tunnel: [_ _ _ _ TRUE _ _] -> w416
      tunnel: [_ _ _ _ _ -1 _] -> w414
      tunnel: [w426 w470 w487 w498 w515 w520 w528] -> w413
      tunnel: w412 -> [w439 w459 w489 w499 w515 w520 _]
      tunnel: [w425 w469 w486 w497 w513 w518 w526] -> w411
      tunnel: w410 -> [w437 w458 w488 _ w513 w518 _]
      tunnel: [w424 w456 w485 w496 w514 w519 w527] -> w409
      tunnel: w408 -> [w424 w456 w485 w495 w514 w519 _]
      tunnel: w407 -> [w423 w449 _ _ _ _ _]
      frame "idle", Default {
        n179 = call "SL2_AD_DLL_Phoibos_GetDeviceState.vi"("dll_path"=w439, "pHandle_in"=w424, "dev_type"=DEF_dev_type."devA (analyzer)", "error in"=w437) -> ("path out"=w436:path, "state"=→"state":T1, "error out"=w435:errorcluster)  [unwired: 2 in]
        n180 = for {
          tunnel: w436 -> [w446]
          tunnel: w424 -> [w445]
          tunnel: w423 -> [w443] mode=indexing
          tunnel: [w442] -> w434 mode=indexing
          tunnel: [w441] -> w426
          shift-right: [w440] -> w425
          shift-left: w435 -> [w444]
          n181 = call "SL2_AD_DLL_Phoibos_GetVoltage.vi"("error in"=w444, "voltage_name"=w443, "pHandle"=w445, "dll path in"=w446) -> ("error out"=w440:errorcluster, "value"=w442:dbl, "dll path out"=w441:path)  [unwired: 3 in]
        }
        n182 = Index Array(array=w434) -> (element #1=→"phoib_I_1":dbl, element #2=→"phoib_I_2":dbl, element #3=→"phoib_I_3":dbl, element #4=→"phoib_I_4":dbl, element #5=→"phoib_I_5":dbl, element #6=→"phoib_I_6":dbl)  [unwired: 6 in]
      }
      frame "set" {
        n183 = Dequeue Element(queue=w468) -> ()  [unwired: 2 in, 4 out]
        n184 = Multiply(x="VoltageRange", y=13) -> (x*y=w465:i32)
        n185 = Add(x="Mode", y=w465) -> (x+y=w462:i32)
        n186 = Build Array("phoib_I_1s", "phoib_I_2s", "phoib_I_3s", "phoib_I_4s", "phoib_I_5s", "phoib_I_6s") -> (w448:dbl[])
        n187 = Index Array(array=u32[] [251749632, 251749633, 251749634, 251749635, 251749636, 251749637, 251749638, 251749639, 251749640, 251749641, 251749642, 251749643, 251749644, 251749645, 251749646, 251749647, 251749648, 251749649, 251749650, 251749651, 251749652, 251749653, 251749654, 251749655, 251749656, 251749657, 251749658, 251749659, 251749660, 251749661, 251749662, 251749663, 251749664, 251749665, 251749666, 251749667, 251749668, 251749669, 251749670, 251749671, 251749672, 251749673, 251749674, 251749675, 251749676, 251749677, 251749678, 251749679, 251749680, 251749681, 251749682, 251749683, 251749684, 251749685, 251749686, 251749687, 251749688, 251749689, 251749690, 251749691, 251749692, 251749693, 251749694, 251749695, 251749696] ("modeIDs"), index=w462) -> (element=w460:u32)
        n188 = call "SL2_AD_DLL_Phoibos_SetDeviceMode.vi"("pHandle"=w456, "error in"=w458, "value"=w460, "dev_type"=DEF_dev_type."devA (analyzer)", "dll path in"=w459) -> ("error out"=w447:errorcluster, "dll path out"=w457:path)  [unwired: 4 in]
        n189 = for {
          tunnel: w456 -> [w476]
          shift-right: [w483] -> w470
          shift-left: w457 -> [w480]
          tunnel: w449 -> [w475] mode=indexing
          tunnel: w448 -> [w474] mode=indexing
          shift-right: [w482] -> w469
          shift-left: w447 -> [w478]
          n190 = call "SL2_AD_DLL_Phoibos_GetVoltageRange.vi"("error in"=w478, "voltage_name"=w475, "pHandle"=w476, "dll path in"=w480) -> ("error out"=w477:errorcluster, "min"=w472:dbl, "max"=w473:dbl, "dll path out"=w479:path)  [unwired: 2 in]
          n191 = In Range and Coerce(upper limit=w473, x=w474, lower limit=w472) -> (coerced(x)=w471:dbl)  [unwired: 1 out]
          n192 = call "SL2_AD_DLL_Phoibos_SetVoltage.vi"("commit"=TRUE, "pHandle"=w476, "error in"=w477, "value"=w471, "voltageName"=w475, "dll path in"=w479) -> ("error out"=w482:errorcluster, "dll path out"=w483:path)  [unwired: 3 in]
        }
      }
      frame "standby" {
        w490 = T1 0 items=["Off"=-1, "Standby"=0, "On"=1] ("state")
        n193 = Dequeue Element(queue=w484) -> ()  [unwired: 2 in, 4 out]
        n194 = call "SL2_AD_DLL_Phoibos_SetDeviceState.vi"("pHandle_in"=w485, "error in"=w488, "state"=w490, "dev_type"=DEF_dev_type."devA (analyzer)", "dll_path"=w489) -> ("error out"=w486:errorcluster, "path out"=w487:path)  [unwired: 2 in]
      }
      frame "release" {
        n195 = Dequeue Element(queue=w500) -> ()  [unwired: 2 in, 4 out]
        n196 = flat-sequence {
          tunnel: w499 -> [w508]
          tunnel: w495 -> [w501]
          tunnel: [w507] -> w494
          tunnel: [w506] -> w493
          tunnel: [u32 0] -> w492
          tunnel: [w510] -> w496
          tunnel: [w511] -> w497
          tunnel: [w512] -> w498
          tunnel: w494 -> [w512]
          tunnel: w493 -> [w511]
          tunnel: w492 -> [w510]
          frame #0 {
            w503 = T1 -1 items=["Off"=-1, "Standby"=0, "On"=1] ("state")
            n197 = call "SL2_AD_DLL_Phoibos_SetDeviceState.vi"("pHandle_in"=w501, "state"=w503, "dev_type"=DEF_dev_type."devA (analyzer)", "dll_path"=w508) -> ("path out"=w502:path)  [unwired: 3 in, 1 out]
            n198 = call "SL2_AD_DLL_Phoibos_Shutdown.vi"("pHandle"=w501, "dll path in"=w502) -> ("error out"=w506:errorcluster, "dll path out"=w507:path)  [unwired: 4 in]
          }
          frame #1 {
            n199 = local write "phoib_con?"(FALSE ("phoib_con?")) -> ()
          }
        }
      }
      frame "close" {
        n200 = Release Queue(queue=w517) -> ()  [unwired: 2 in, 3 out]
      }
      frame "suspend" {
        n201 = Dequeue Element(queue=w521) -> ()  [unwired: 2 in, 4 out]
      }
      frame "init" {
        n202 = Dequeue Element(queue=w529) -> ()  [unwired: 2 in, 4 out]
        n203 = flat-sequence {
          tunnel: [w532] -> w525
          tunnel: [w533] -> w524
          tunnel: [w534] -> w523
          tunnel: [w547] -> w526
          tunnel: [w548] -> w527
          tunnel: [w549] -> w528
          tunnel: w525 -> [w549]
          tunnel: w524 -> [w547]
          tunnel: w523 -> [w548]
          frame #0 {
            n204 = local write "phoib_con?"(FALSE ("phoib_con?")) -> ()
          }
          frame #1 {
            n205 = call "GetSL2AD_VI_dllPath.vi"() -> ("error"=w543:errorcluster, "Path"=w544:path)  [unwired: 9 in, 1 out]
            n206 = call "SL2_AD_DLL_List_Devices.vi"("error in"=w543, "dev_type"=DEF_dev_type."devA (analyzer)", "dll path in"=w544) -> ("error out"=w538:errorcluster, "devices"=w542:string[], "dll path out"=w539:path)  [unwired: 2 in]
            n207 = Index Array(array=w542, index=0) -> (element=w540:string)
            n208 = call "SL2_AD_DLL_Phoibos_Initialize.vi"("error in"=w538, "detectorId"="", "analyzerId"=w540, "dll_path"=w539) -> ("error out"=w535:errorcluster, "pHandle"=w534:u32, "path out"=w536:path)  [unwired: 1 in]
            n209 = call "SL2_AD_DLL_Phoibos_ListDeviceModes.vi"("dll path in"=w536, "dev_type"=DEF_dev_type."devA (analyzer)", "pHandle"=w534, "error in"=w535) -> ("dll path out"=w532:path, "error out"=w533:errorcluster)  [unwired: 1 in, 2 out]
          }
          frame #2 {
            n210 = local write "phoib_con?"(TRUE ("phoib_con?")) -> ()
          }
        }
      }
    }
    "error out 2" <- w411
  }
